vi "End Effector Motor Control.vi"(10 "Analog Input (closing)":dbl, 11 "Analog Input (opening)":dbl) -> ()   [LabVIEW 2014]
uses:
  <vilib>/Rock Robotics/WPI/Joystick/WPI_JoystickGetSetRefNum.vi
  <vilib>/Rock Robotics/Network Tables/SD Write Number.vi
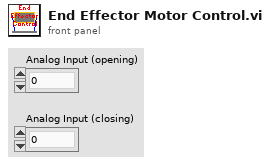
[diagram p1: front panel]
types:
  T1 = typedef "WPI_SwitchDevRef.ctl" = cluster{"DevStatus":errorcluster, "DIO Channel":T2, "Controller":T3, "CntIndex":T4, "Normally Closed":bool}
  T2 = typedef "FPGA_DIOChannel.ctl" = enum8{"DIO 0", "DIO 1", "DIO 2", "DIO 3", "DIO 4", "DIO 5", "DIO 6", "DIO 7", "DIO 8", "DIO 9", "DIO MXP 0", "DIO MXP 1", "DIO MXP 2", "DIO MXP 3", "DIO MXP 4", "DIO MXP 5", "DIO MXP 6", "DIO MXP 7", "DIO MXP 8", "DIO MXP 9", "DIO MXP 10", "DIO MXP 11", "DIO MXP 12", "DIO MXP 13", "DIO MXP 14", "DIO MXP 15", "Invalid"}
  T3 = typedef "FPGA_TypedefDigitalModule.ctl" = enum16{"Controller 1"}
  T4 = typedef "FPGA_CounterCtrSystemIndex.ctl" = enum8{"Ctr 0", "Ctr 1", "Ctr 2", "Ctr 3", "Ctr 4", "Ctr 5", "Ctr 6", "Ctr 7", "Invalid"}
  T5 = typedef "WPI_JoystickDevRef.ctl" = cluster{"Device":T6}
  T6 = typedef "WPI_JoystickDeviceEnum.ctl" = enum16{"USB 0", "USB 1", "USB 2", "USB 3", "USB 4", "USB 5"}
  T7 = typedef "WPI_MotorControlDeviceRef.ctl" = cluster{"DeviceStatus":errorcluster, "Type":T8, "PWM":cluster{"Controller":T3, "PWM Channel":T9, "DeadBand":T10}, "CAN":cluster{"Device Number":u8, "Control Mode":T11, "Semaphore":T12, "Max Vout":dbl, "TalonSRX Control Mode":T13}, "Invert":bool, "TransformRef":T14, "InvTransformRef":T14}
  T8 = typedef "WPI_MotorControlType.ctl" = enum16{"PWM", "CAN", "CANTalonSRX"}
  T9 = typedef "FPGA_DIOPWMChannel.ctl" = enum8{"PWM 0", "PWM 1", "PWM 2", "PWM 3", "PWM 4", "PWM 5", "PWM 6", "PWM 7", "PWM 8", "PWM 9", "PWM MXP 0", "PWM MXP 1", "PWM MXP 2", "PWM MXP 3", "PWM MXP 4", "PWM MXP 5", "PWM MXP 6", "PWM MXP 7", "PWM MXP 8", "PWM MXP 9", "Invalid"}
  T10 = typedef "WPI_PWMDeadband.ctl" = cluster{"Name":string, "maxPositivePwm":i32, "minPositivePwm":i32, "centerPwm":i32, "maxNegativePwm":i32, "minNegativePwm":i32, "angularRange":u16}
  T11 = typedef "WPI_CANJaguar_ControlMode.ctl" = enum8{"Percent VBus", "Current", "Speed", "Position", "Voltage"}
  T12 = typedef "Semaphore RefNum" = refnum<k1>
  T13 = typedef "WPI_CANTalonSRX_APIControlMode.ctl" = enum8{"Percent VBus", "Speed", "Position", "Slave", "Unchanged / Invalid"}
  T14 = typedef "WPI_PWMTransform_ConPane.ctl" = refnum<vi>
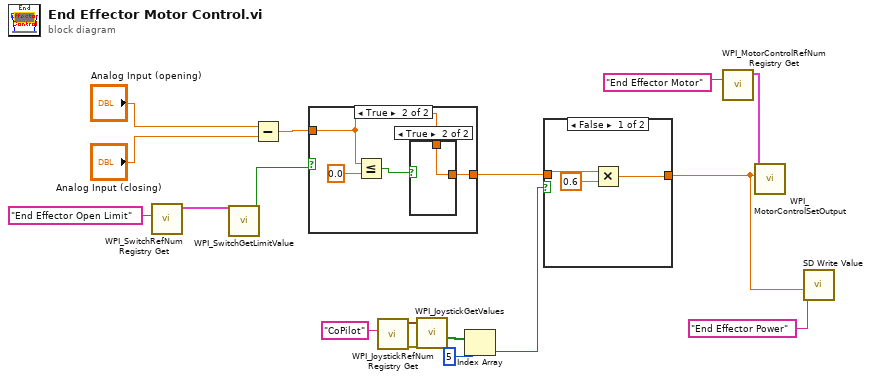
[diagram p0: block diagram]
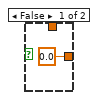
[diagram p4: hidden frame]
diagram:
  n1 = call <vilib>:"WPI_SwitchRefNum Registry Get.vi"("refnum name"="End Effector Open Limit") -> ("SwitchDevRef"=w17:T1)  [unwired: 9 in, 1 out]
  n2 = call <vilib>:"WPI_SwitchGetLimitValue.vi"("SwitchDevRef"=w17) -> ("Switch Pressed"=w13:bool)  [unwired: 8 in, 2 out]
  n3 = Subtract(x="Analog Input (opening)", y="Analog Input (closing)") -> (x-y=w10:dbl)
  n4 = case shown="True" w13 {
    tunnel: w10 -> [w18 w19]
    tunnel: [w18 w20] -> w3
    frame False {
    }
    frame True {
      n5 = Less Or Equal?(x=w19, y=0.0) -> (x <= y?=w21:bool)
      n6 = case shown="True" w21 {
        tunnel: [0.0 w24] -> w20
        tunnel: w19 -> [_ w24]
        frame False {
        }
        frame True {
        }
      }
    }
  }
  n7 = call <vilib>:"WPI_JoystickRefNum Registry Get.vi"("refnum name"="CoPilot") -> ("error out"=w9:errorcluster, "JoystickDevRef"=w8:T5)  [unwired: 9 in]
  n8 = call <vilib>:"WPI_JoystickGetValues.vi"("error in (no error)"=w9, "JoystickDevRef"=w8) -> ("Buttons"=w6:bool[])  [unwired: 5 in, 4 out]
  n9 = Index Array(array=w6, index=5) -> (element=w4:bool)
  n10 = case shown="False" w4 {
    tunnel: w3 -> [w27 w28]
    tunnel: [w26 w28] -> w1
    frame False {
      n11 = Multiply(x=w27, y=0.6) -> (x*y=w26:dbl)
    }
    frame True {
    }
  }
  n12 = call <vilib>:"WPI_MotorControlRefNum Registry Get.vi"("refnum name"="End Effector Motor") -> ("MotorControlDevRef"=w14:T7)  [unwired: 9 in, 1 out]
  n13 = call <vilib>:"WPI_MotorControlSetOutput.vi"("Output"=w1, "MotorControlDevRef"=w14) -> ()  [unwired: 7 in, 3 out]
  n14 = call-poly <vilib>:"SD Write Value.vi"("Numeric"=w1, "Name"="End Effector Power") -> ()  [unwired: 8 in, 2 out]
